vi "probe_tool.vi"() -> ()   [LabVIEW 2020]
panel:
  in  "stop":bool
  in  "Click to write":bool=TRUE caption="Enable"
  out "Slide 2":u8(slide) scale=0.0..100.0
  in  "Slide":dbl(slide) scale=0.0..10.0
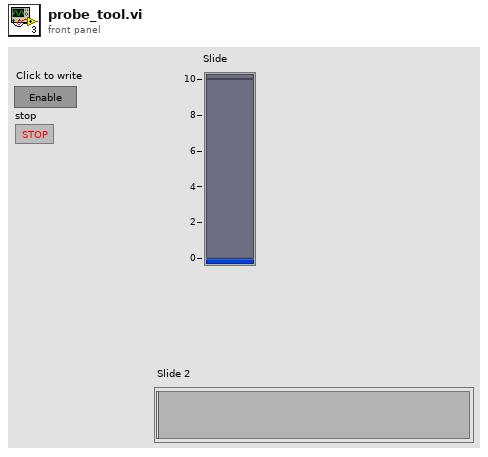
[diagram p1: front panel]
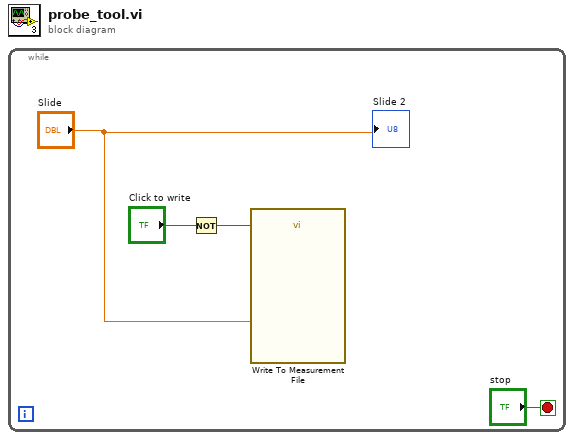
[diagram p0: block diagram]
diagram:
  n1 = while {
    stop <- "stop" stop-if-true
    n2 = Not(x="Click to write") -> (.not. x?=w3:bool)
    n3 = call "Write To Measurement File"("Signals"="Slide", "Enable"=w3) -> ()  [unwired: 15 in, 3 out]
    "Slide 2" <- "Slide"
  }
